vi "SCP Close.vi"(8 "Error In":errorcluster, 11 "SCP Session":refnum<k24>) -> (0 "Error Out":errorcluster)   [LabVIEW 2020, in "LMH-LINX.lvlib"]
uses:
  LMH-LINX.lvlib
  c:/p4/penguin/lvaddon/MakerHub/LINX/trunk/20.1/objects/MakerHub_LINX/win32U/i386/msvc90/release/LabVIEW/vi.lib/MakerHub/LINX/Resources/Renci.SshNet.dll
  Resources/Renci.SshNet.dll
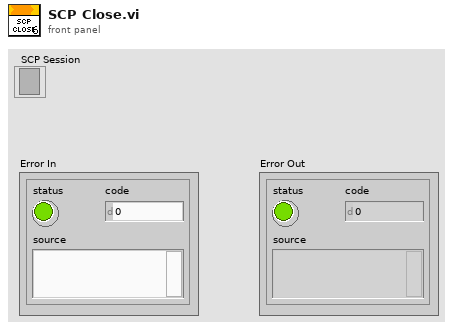
[diagram p1: front panel]
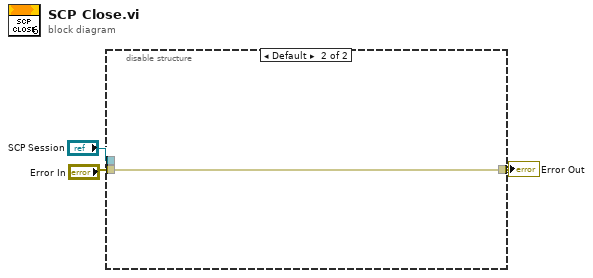
[diagram p0: block diagram]
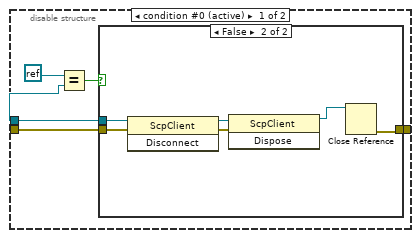
[diagram p2: hidden frame]
diagram:
  n1 = disable-structure shown="Default" {
    disable-tunnel: [w8 w16] -> w3
    disable-tunnel: "Error In" -> [w7 w16]
    disable-tunnel: "SCP Session" -> [w5 _]
    frame condition #0 (active) {
      n2 = Equal?(x=refnum<k0> refnum, y=w5) -> (x = y?=w4:bool)
      n3 = case shown="False" w4 {
        tunnel: [w9 w10] -> w8
        tunnel: w7 -> [w9 w13]
        tunnel: w5 -> [_ w12]
        frame True {
        }
        frame False {
          n4 = invoke class="ScpClient" method="Disconnect"(reference=w12, error in=w13) -> (reference out=w15:refnum<k24>, error out=w14:errorcluster)  [unwired: 1 in, 1 out]
          n5 = invoke class="ScpClient" method="Dispose"(reference=w15, error in=w14) -> (reference out=w11:refnum<k24>)  [unwired: 1 in, 2 out]
          n6 = Close Reference(reference=w11) -> (error out=w10:errorcluster)  [unwired: 1 in]
        }
      }
    }
    frame condition #1 {
    }
  }
  "Error Out" <- w3
